vi "Get Path Regex.vi"(8 "error in (no error)":errorcluster, 11 "PublishConfigController in":refnum<class "PublishConfigController.lvclass">) -> (0 "error out":errorcluster, 2 "Path Regex":string, 3 "PublishConfigController out":refnum<class "PublishConfigController.lvclass">)   [LabVIEW 2020, in "Vecto.lvlib" / "PublishConfigController.lvclass"]
uses:
  PublishConfigController.lvclass
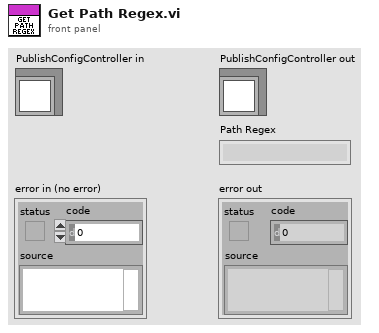
[diagram p1: front panel]
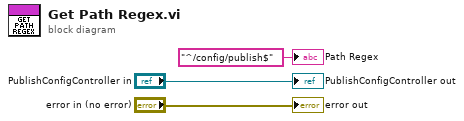
[diagram p0: block diagram]
diagram:
  "error out" <- "error in (no error)"
  "PublishConfigController out" <- "PublishConfigController in"
  "Path Regex" <- "^/config/publish$" ("Path Regex")
